vi "PulseIntervalHistogram.vi"(6 "Last rising flank in":i32, 7 "Last reference value in":bool, 8 "Pulse count in":u64, 9 "No of SI bins":dbl=50.0, 11 "Binary array probe":bool[](array[boolean])) -> (0 "Pulse count out":u64, 1 "Interflank intervals out":i32[](array[numeric]), 2 "Pulse length histogram":T1(graph), 3 "Pulse period histogram":T1(graph), 4 "Last rising flank out":i32, 5 "Last reference value out":bool)   [LabVIEW 2012]
uses:
  <vilib>/Analysis/NI_AALPro.lvlib
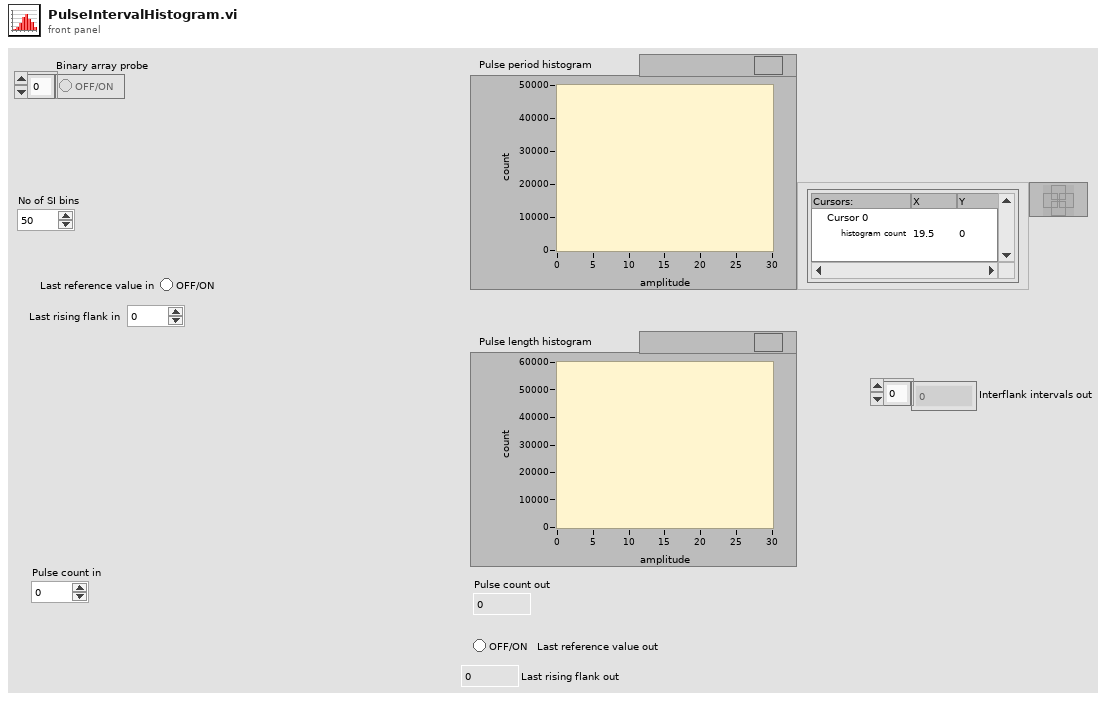
[diagram p1: front panel]
types:
  T1 = cluster{"X Values":dbl[], "Histogram: h(x)":i32[]}
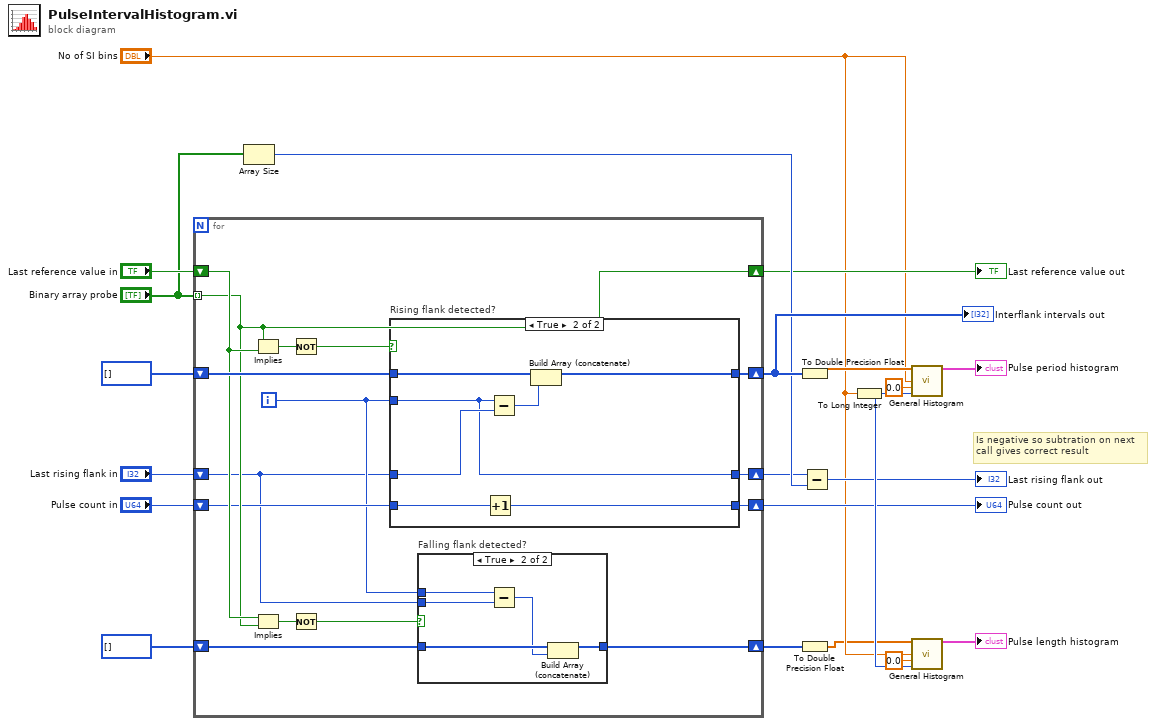
[diagram p0: block diagram]
diagram:
  # "Is negative so subtration on next\ncall gives correct result"
  n1 = for {
    tunnel: "Binary array probe" -> [w30] mode=indexing
    shift-right: [w30] -> w6
    shift-left: "Last reference value in" -> [w31]
    shift-right: [w34] -> w9
    shift-left: "Last rising flank in" -> [w22]
    shift-right: [w33] -> w19
    shift-left: i32[] [] -> [w32]
    shift-right: [w26] -> w16
    shift-left: i32[] [] -> [w27]
    shift-right: [w24] -> w12
    shift-left: "Pulse count in" -> [w25]
    i -> [w23]
    n2 = Implies(1:w31, 2:w30) -> (0:w36:bool)
    n3 = Implies(1:w30, 2:w31) -> (0:w29:bool)
    n4 = Not(x=w36) -> (.not. x?=w35:bool)
    n5 = Not(x=w29) -> (.not. x?=w28:bool)
    n6 = case "Rising flank detected?" shown="True" w35 {
      tunnel: w23 -> [_ w47]
      tunnel: [w43 w47] -> w34
      tunnel: [w45 w52] -> w33
      tunnel: w32 -> [w45 w51]
      tunnel: w25 -> [w44 w50]
      tunnel: [w44 w49] -> w24
      tunnel: w22 -> [w43 w48]
      frame False {
      }
      frame True {
        n7 = Increment(x=w50) -> (x+1=w49:u64)
        n8 = Subtract(x=w47, y=w48) -> (x-y=w46:i32)
        n9 = Build Array (concatenate)(w51, w46) -> (w52:i32[])
      }
    }
    n10 = case "Falling flank detected?" shown="True" w28 {
      tunnel: w27 -> [w37 w41]
      tunnel: w23 -> [_ w42]
      tunnel: [w37 w39] -> w26
      tunnel: w22 -> [_ w38]
      frame False {
      }
      frame True {
        n11 = Subtract(x=w42, y=w38) -> (x-y=w40:i32)
        n12 = Build Array (concatenate)(w41, w40) -> (w39:i32[])
      }
    }
  }
  "Pulse count out" <- w12
  "Last reference value out" <- w6
  "Interflank intervals out" <- w19
  n13 = Array Size(array="Binary array probe") -> (size(s)=w10:i32)
  n14 = To Double Precision Float(number=w19) -> (double precision float=w5:dbl[])
  n15 = To Double Precision Float(number=w16) -> (double precision float=w2:dbl[])
  n16 = Subtract(x=w9, y=w10) -> (x-y=→"Last rising flank out":i32)
  n17 = To Long Integer(number="No of SI bins") -> (32bit integer=w15:i32)
  n18 = call <vilib>:"General Histogram.vi"("X"=w5, "max"="No of SI bins", "min"=0.0, "# bins"=w15) -> ("Histogram Graph"=→"Pulse period histogram":T1)  [unwired: 7 in, 4 out]
  n19 = call <vilib>:"General Histogram.vi"("X"=w2, "max"="No of SI bins", "min"=0.0, "# bins"=w15) -> ("Histogram Graph"=→"Pulse length histogram":T1)  [unwired: 7 in, 4 out]
